vi "wire to tag bus.vi"(8 "error in":errorcluster, 10 "wire data":string, 11 "data table in":T1) -> (0 "error out":errorcluster, 3 "data table out":T1)   [LabVIEW 2013, in "TEC runtime.lvclass"]
uses:
  TEC runtime.lvclass
  <vilib>/NI/Tag Bus/table/data table.ctl
  <vilib>/NI/Tag Bus/table/data table.lvlib
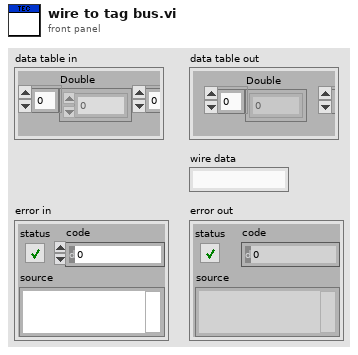
[diagram p1: front panel]
types:
  T1 = typedef "tag bus.lvlib/data table.lvlib/data table.ctl" = cluster{"Double":dbl[], "Single":sgl[], "I64":i64[], "I32":i32[], "I16":i16[], "I8":i8[], "U64":u64[], "U32":u32[], "U16":u16[], "U8":u8[], "Boolean":bool[], "String":string[], "Array of Double":cluster{"DBL Array":dbl[]}[], "Array of Single":cluster{"SGL Array":sgl[]}[], "Array of I64":cluster{"I64 Array":i64[]}[], "Array of I32":cluster{"I32 Array":i32[]}[], "Array of I16":cluster{"I16 Array":i16[]}[], "Array of I8":cluster{"I8 Array":i8[]}[], "Array of U64":cluster{"U64 Array":u64[]}[], "Array of U32":cluster{"U32 Array":u32[]}[], "Array of U16":cluster{"U16 Array":u16[]}[], "Array of U8":cluster{"U8 Array":u8[]}[], "Array of Boolean":cluster{"Boolean Array":bool[]}[], "Array of String":cluster{"String Array":string[]}[]}
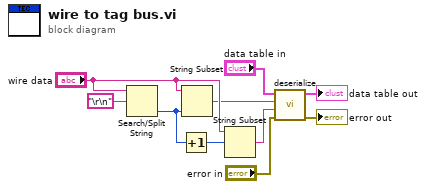
[diagram p0: block diagram]
diagram:
  n1 = Search/Split String(string="wire data", search string/char (-)="\r\n") -> (offset of match=w9:i32)  [unwired: 1 in, 2 out]
  n2 = Increment(x=w9) -> (x+1=w8:i32)
  n3 = String Subset(string="wire data", length (rest)=w9) -> (substring=w6:string)  [unwired: 1 in]
  n4 = String Subset(string="wire data", offset (0)=w8) -> (substring=w5:string)  [unwired: 1 in]
  n5 = call <vilib>:"deserialize.vi"("error in"="error in", "data"=w5, "version"=w6, "data table in"="data table in") -> ("error out"=→"error out":errorcluster, "data table out"=→"data table out":T1)  [unwired: 6 in]
